vi "SS2 Live_Init Settings.vi"(8 "error in (no error)":errorcluster) -> (0 "error out":errorcluster)   [LabVIEW 2019]
uses:
  SS2 Live_Settings List.ctl
  SS2 Gate Configuration.ctl
  SS2 Gate Definition.ctl
  SS2 Live_Gate Configuration Action.ctl
  SS2 Live_File Information.ctl
  SS2 Live_Image ROI Information.ctl
  Phasor/Image Binning Options.ctl
  SS2 DAQ Parameters 3.ctl
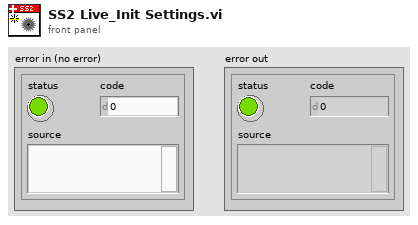
[diagram p1: front panel]
types:
  T1 = typedef "SS2 Gate Configuration.ctl" = cluster{"Gate Configuration":string, "Gate Offset":u32, "Gate Definition":T2}
  T2 = typedef "SS2 Gate Definition.ctl" = cluster{"gs_psincdec_0":u32, "gs_psincdec_1":u32, "gs_psincdec_2":u32, "gs_psincdec_3":u32, "gs_no_shift_adj_1":u32, "gs_no_shift_adj_2":u32, "gs_no_shift_adj_3":u32}
  T3 = typedef "SS2 Live_Settings List.ctl" = enum16{"FPGA:Bitfile Path", "FPGA:Bitfile Version", "FPGA:Auto Reset FPGA", "Acquisition Parameters:SS2 DAQ Parameters", "Acquisition Parameters:Gate Configuration Array", "Acquisition Parameters:Buffer Size (# Gates)", "File Information:File Information", "File Information:# Datasets in Series", "File Information:Scrambled File Flag", "File Information:Delay between Datasets", "Image Parameters:Image ROI Information", "Image Parameters:Image Binning Options", "UI Settings:Histogram Bins Number"}
  T4 = typedef "SS2 Live_Gate Configuration Action.ctl" = enum16{"Get Gate Configuration Name", "Get Configuration by Name", "Add Gate Configuration", "Delete Gate Configuration", "Rename Gate Configuration"}
  T5 = typedef "SS2 Live_File Information.ctl" = cluster{"File Folder":path, "File Name":string, "File Index":u32, "Author":string, "Sample":string, "Compression":bool, "Compression Level":u8}
  T6 = typedef "SS2 Live_Image ROI Information.ctl" = cluster{"Save ROI Only":bool, "Left":u16, "Top":u16, "Right":u16, "Bottom":u16, "Use Current ROI":bool}
  T7 = typedef "Image Binning Options.ctl" = cluster{"Use Image Binning":bool, "X Bin":i32, "Y Bin":i32}
  T8 = typedef "SS2 DAQ Parameters 3.ctl" = cluster{"10 bits":bool, "# Exposure Sequences":u32, "# 1-bit Frame per Gate":u32, "Gate Shift":u32, "# Gates per Set":u32, "# Sets":u32, "Laser Period":dbl[unit], "Sync Period":dbl[unit], "Gate Offset":u32, "Auto-adjust Gate Offset":bool, "Gate Definition":T2}
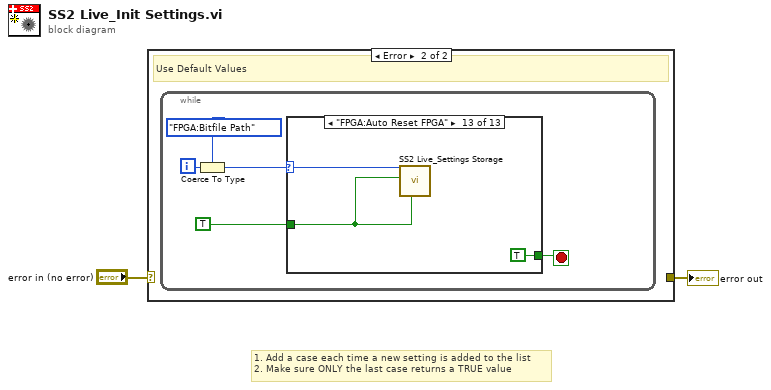
[diagram p0: block diagram]
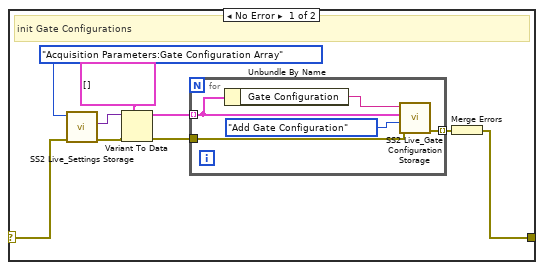
[diagram p2: hidden frame]
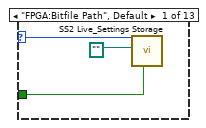
[diagram p3: hidden frame]
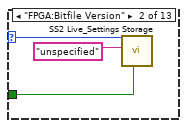
[diagram p4: hidden frame]
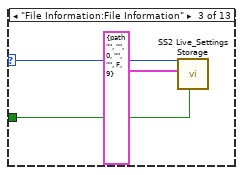
[diagram p5: hidden frame]
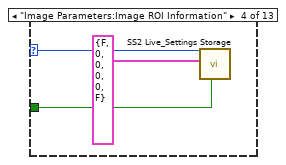
[diagram p6: hidden frame]
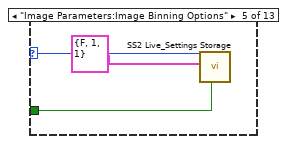
[diagram p7: hidden frame]
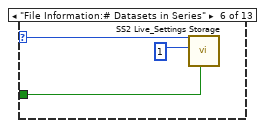
[diagram p8: hidden frame]
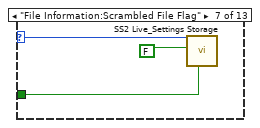
[diagram p9: hidden frame]
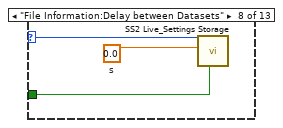
[diagram p10: hidden frame]
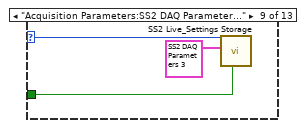
[diagram p11: hidden frame]
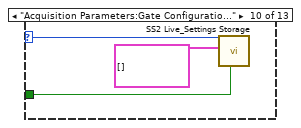
[diagram p12: hidden frame]
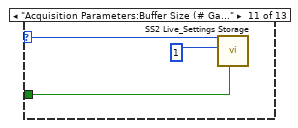
[diagram p13: hidden frame]
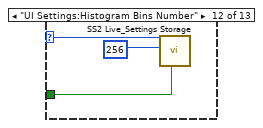
[diagram p14: hidden frame]
diagram:
  # "1. Add a case each time a new setting is added to the list\n2. Make sure ONLY the last case returns a TRUE value"
  n1 = case shown="Error" "error in (no error)" {
    selector: "error in (no error)" -> [w4 _]
    tunnel: [w3 _] -> w1
    frame No Error {
      # "init Gate Configurations"
      n2 = call "SS2 Live_Settings Storage.vi"("Error In"=w4, "Settings List"=SS2_Live_Settings_List."Acquisition Parameters:Gate Configuration Array") -> ("Error Out"=w10:errorcluster, "Variant Data out"=w9:variant)  [unwired: 8 in]
      n3 = Variant To Data(error in=w10, type=T1[] [] ("Gate Configuration Definitions"), Variant=w9) -> (data=w7:T1[], error out=w6:errorcluster)
      n4 = for {
        tunnel: w7 -> [w15] mode=indexing
        tunnel: w6 -> [w13]
        tunnel: [w12] -> w5 mode=indexing
        n5 = Unbundle By Name(w15) -> ("Gate Configuration"=w16:string)
        n6 = call "SS2 Live_Gate Configuration Storage.vi"("Error In"=w13, "Action"=SS2_Live_Gate_Configuration_Action."Add Gate Configuration", "Gate Configuration Definition in"=w15, "Gate Configuration Name in"=w16) -> ("Error Out"=w12:errorcluster)  [unwired: 2 in, 5 out]
      }
      n7 = Merge Errors(w5) -> (w3:errorcluster)
    }
    frame Error {
      # "Use Default Values"
      n8 = while {
        i -> [w21]
        stop <- w17 stop-if-true
        n9 = Coerce To Type(0:w21, 1:SS2_Live_Settings_List."FPGA:Bitfile Path" ("Settings List")) -> (2:w19:T3)
        n10 = case shown="\"FPGA:Auto Reset FPGA\"" w19 {
          selector: w19 -> [w24 w27 w30 w33 w36 w39 w42 w45 w48 w51 w54 w57 w60]
          tunnel: TRUE -> [w23 w26 w29 w32 w35 w38 w41 w44 w47 w50 w53 w56 w58]
          tunnel: [_ _ _ _ _ _ _ _ _ _ _ _ TRUE] -> w17
          frame "FPGA:Bitfile Path", Default {
            n11 = call "SS2 Live_Settings Storage.vi"("Set/Get(F)"=w23, "Variant Data in"=path "", "Settings List"=w24) -> ()  [unwired: 7 in, 2 out]
          }
          frame "FPGA:Bitfile Version" {
            n12 = call "SS2 Live_Settings Storage.vi"("Set/Get(F)"=w26, "Variant Data in"="unspecified", "Settings List"=w27) -> ()  [unwired: 7 in, 2 out]
          }
          frame "File Information:File Information" {
            n13 = call "SS2 Live_Settings Storage.vi"("Set/Get(F)"=w29, "Variant Data in"=T5 {"File Folder"=path "", "File Name"="", "File Index"=0, "Author"="", "Sample"="", "Compression"=FALSE, "Compression Level"=9} ("File Information"), "Settings List"=w30) -> ()  [unwired: 7 in, 2 out]
          }
          frame "Image Parameters:Image ROI Information" {
            n14 = call "SS2 Live_Settings Storage.vi"("Set/Get(F)"=w32, "Variant Data in"=T6 {"Save ROI Only"=FALSE, "Left"=0, "Top"=0, "Right"=0, "Bottom"=0, "Use Current ROI"=FALSE} ("Image Information"), "Settings List"=w33) -> ()  [unwired: 7 in, 2 out]
          }
          frame "Image Parameters:Image Binning Options" {
            n15 = call "SS2 Live_Settings Storage.vi"("Set/Get(F)"=w35, "Variant Data in"=T7 {"Use Image Binning"=FALSE, "X Bin"=1, "Y Bin"=1} ("Image Binning Options"), "Settings List"=w36) -> ()  [unwired: 7 in, 2 out]
          }
          frame "File Information:# Datasets in Series" {
            n16 = call "SS2 Live_Settings Storage.vi"("Set/Get(F)"=w38, "Variant Data in"=1, "Settings List"=w39) -> ()  [unwired: 7 in, 2 out]
          }
          frame "File Information:Scrambled File Flag" {
            n17 = call "SS2 Live_Settings Storage.vi"("Set/Get(F)"=w41, "Variant Data in"=FALSE, "Settings List"=w42) -> ()  [unwired: 7 in, 2 out]
          }
          frame "File Information:Delay between Datasets" {
            w43 = dbl[unit] 0.0  # s
            n18 = call "SS2 Live_Settings Storage.vi"("Set/Get(F)"=w44, "Variant Data in"=w43, "Settings List"=w45) -> ()  [unwired: 7 in, 2 out]
          }
          frame "Acquisition Parameters:SS2 DAQ Parameters" {
            n19 = call "SS2 Live_Settings Storage.vi"("Set/Get(F)"=w47, "Variant Data in"=T8 {"10 bits"=FALSE, "# Exposure Sequences"=100, "# 1-bit Frame per Gate"=255, "Gate Shift"=0, "# Gates per Set"=1, "# Sets"=1, "Laser Period"=0.0, "Sync Period"=0.0, "Gate Offset"=650, "Auto-adjust Gate Offset"=FALSE, "Gate Definition"={"gs_psincdec_0"=1, "gs_psincdec_1"=0, "gs_psincdec_2"=0, "gs_psincdec_3"=0, "gs_no_shift_adj_1"=65, "gs_no_shift_adj_2"=90, "gs_no_shift_adj_3"=30}} ("SS2 DAQ Parameters"), "Settings List"=w48) -> ()  [unwired: 7 in, 2 out]
          }
          frame "Acquisition Parameters:Gate Configuration Array" {
            n20 = call "SS2 Live_Settings Storage.vi"("Set/Get(F)"=w50, "Variant Data in"=T1[] [] ("Gate Configuration Definitions"), "Settings List"=w51) -> ()  [unwired: 7 in, 2 out]
          }
          frame "Acquisition Parameters:Buffer Size (# Gates)" {
            n21 = call "SS2 Live_Settings Storage.vi"("Set/Get(F)"=w53, "Variant Data in"=u32 1 ("Buffer Size #Gates)"), "Settings List"=w54) -> ()  [unwired: 7 in, 2 out]
          }
          frame "UI Settings:Histogram Bins Number" {
            n22 = call "SS2 Live_Settings Storage.vi"("Set/Get(F)"=w56, "Variant Data in"=256, "Settings List"=w57) -> ()  [unwired: 7 in, 2 out]
          }
          frame "FPGA:Auto Reset FPGA" {
            n23 = call "SS2 Live_Settings Storage.vi"("Set/Get(F)"=w58, "Variant Data in"=w58, "Settings List"=w60) -> ()  [unwired: 7 in, 2 out]
          }
        }
      }
    }
  }
  "error out" <- w1
